vi "Read Element of Glue Resivoir Slots.vi"(8 "error in (no error)":errorcluster, 10 "index":i32, 11 "WorkTable Class in":refnum<class "WorkTable Class.lvclass">) -> (0 "error out":errorcluster, 2 "Glue Resivoir Slot":T1, 3 "WorkTable Class out":refnum<class "WorkTable Class.lvclass">)   [LabVIEW 2011, in "WorkTable Class.lvclass"]
uses:
  WorkTable Class.lvclass
  WorkTable Class.lvclass/WorkTable Class.ctl
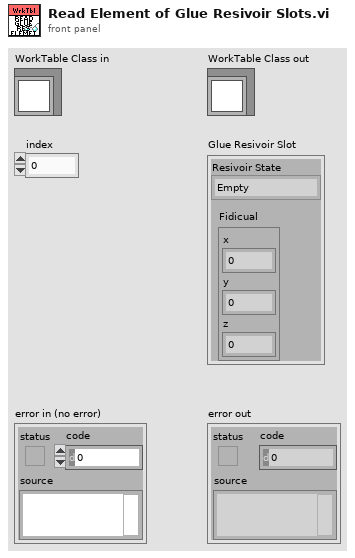
[diagram p1: front panel]
types:
  T1 = cluster{"Resivoir State":enum16{"Empty", "Full", "Used"}, "Fidicual ":cluster{"x":dbl, "y":dbl, "z":dbl}}
  T2 = cluster{"Resivoir State":enum16{"Empty", "Full", "Used"}, "Fidicual ":cluster{"x":dbl, "y":dbl, "z":dbl}}[]
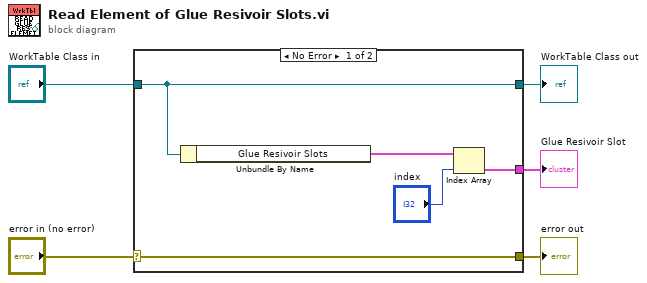
[diagram p0: block diagram]
diagram:
  n1 = case shown="No Error" "error in (no error)" {
    selector: "error in (no error)" -> [w10 w11]
    tunnel: [w10 w11] -> w4
    tunnel: [w9 w12] -> w2
    tunnel: "WorkTable Class in" -> [w9 w12]
    tunnel: [w6 _] -> w1
    frame No Error {
      n2 = Unbundle By Name(w9) -> ("Glue Resivoir Slots"=w8:T2)
      n3 = Index Array(array=w8, index="index") -> (element=w6:T1)
    }
    frame Error {
    }
  }
  "error out" <- w4
  "WorkTable Class out" <- w2
  "Glue Resivoir Slot" <- w1
